vi "Set Target Frequency.vi"(8 "Error In":errorcluster, 10 "Target Frequency":dbl, 11 "TimerDRV in":refnum<class "TimerDRV.lvclass">) -> (0 "Error Out":errorcluster, 3 "TimerDRV out":refnum<class "TimerDRV.lvclass">)   [LabVIEW 2019, in "TimingDRV Engine.lvlib" / "TimerDRV.lvclass"]
uses:
  TimerDRV.lvclass
  TimerDRV.lvclass/TimerDRV.ctl
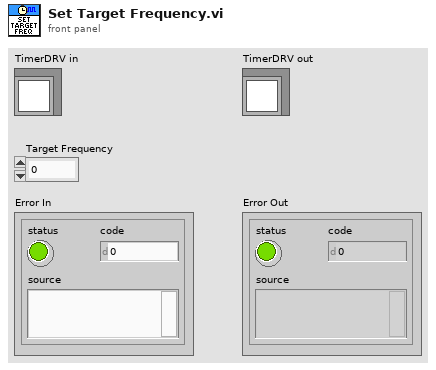
[diagram p1: front panel]
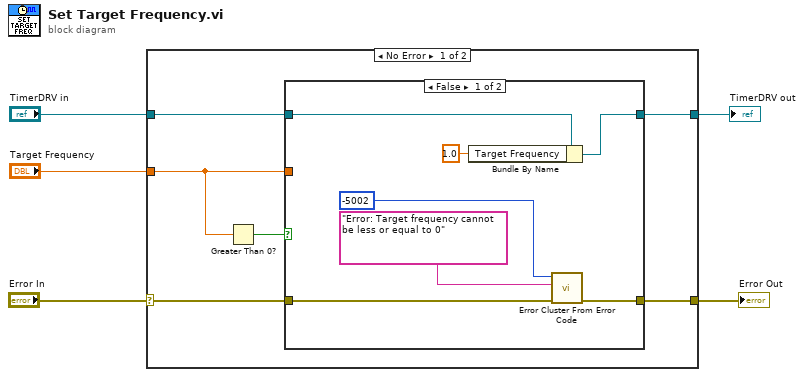
[diagram p0: block diagram]
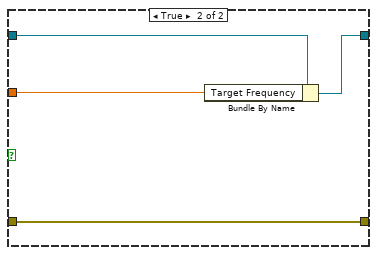
[diagram p2: hidden frame]
diagram:
  n1 = case shown="No Error" "Error In" {
    selector: "Error In" -> [w7 w24]
    tunnel: "TimerDRV in" -> [w11 w23]
    tunnel: [w10 w23] -> w4
    tunnel: "Target Frequency" -> [w9 _]
    tunnel: [w6 w24] -> w1
    frame No Error {
      n2 = Greater Than 0?(x=w9) -> (x > 0?=w8:bool)
      n3 = case shown="False" w8 {
        tunnel: w11 -> [w18 w22]
        tunnel: [w14 w21] -> w10
        tunnel: w9 -> [_ w20]
        tunnel: w7 -> [w17 w19]
        tunnel: [w13 w19] -> w6
        frame False {
          n4 = Bundle By Name(cluster=w18, "Target Frequency"=1.0) -> (w14:refnum<class "TimerDRV.lvclass">)
          n5 = call <vilib>:"Error Cluster From Error Code.vi"("error in (no error)"=w17, "error message (\"\")"="Error: Target frequency cannot be less or equal to 0" ("error message (\"\")"), "error code (0)"=-5002) -> ("error out"=w13:errorcluster)  [unwired: 6 in]
        }
        frame True {
          n6 = Bundle By Name(cluster=w22, "Target Frequency"=w20) -> (w21:refnum<class "TimerDRV.lvclass">)
        }
      }
    }
    frame Error {
    }
  }
  "TimerDRV out" <- w4
  "Error Out" <- w1
